vi "Configure.vi"(8 "error in (no error)":errorcluster, 9 "Path":path, 10 "Interactive?":bool, 11 "XML Report In":refnum<class "XML Report.lvclass">) -> (0 "error out":errorcluster, 3 "XML Report Out":refnum<class "XML Report.lvclass">)   [LabVIEW 2020, in "XML Report.lvclass"]
uses:
  XML Report.lvclass
  XML Report.lvclass/XML Report.ctl
  Framework/Configuration Manager/Configuration Manager.lvclass
panel:
  in  "Cancel":bool
  in  "Commit":bool
  in  "Open New Reports":bool
  in  "Report Path":path
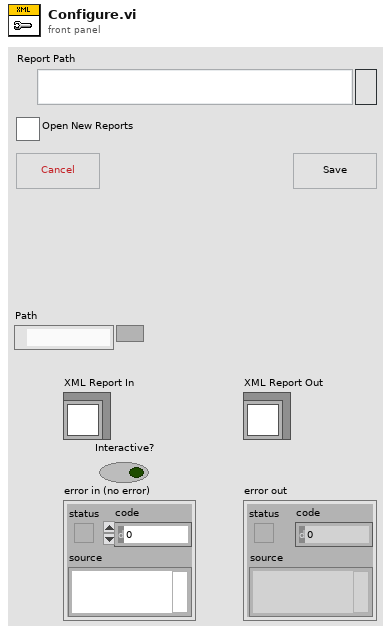
[diagram p1: front panel]
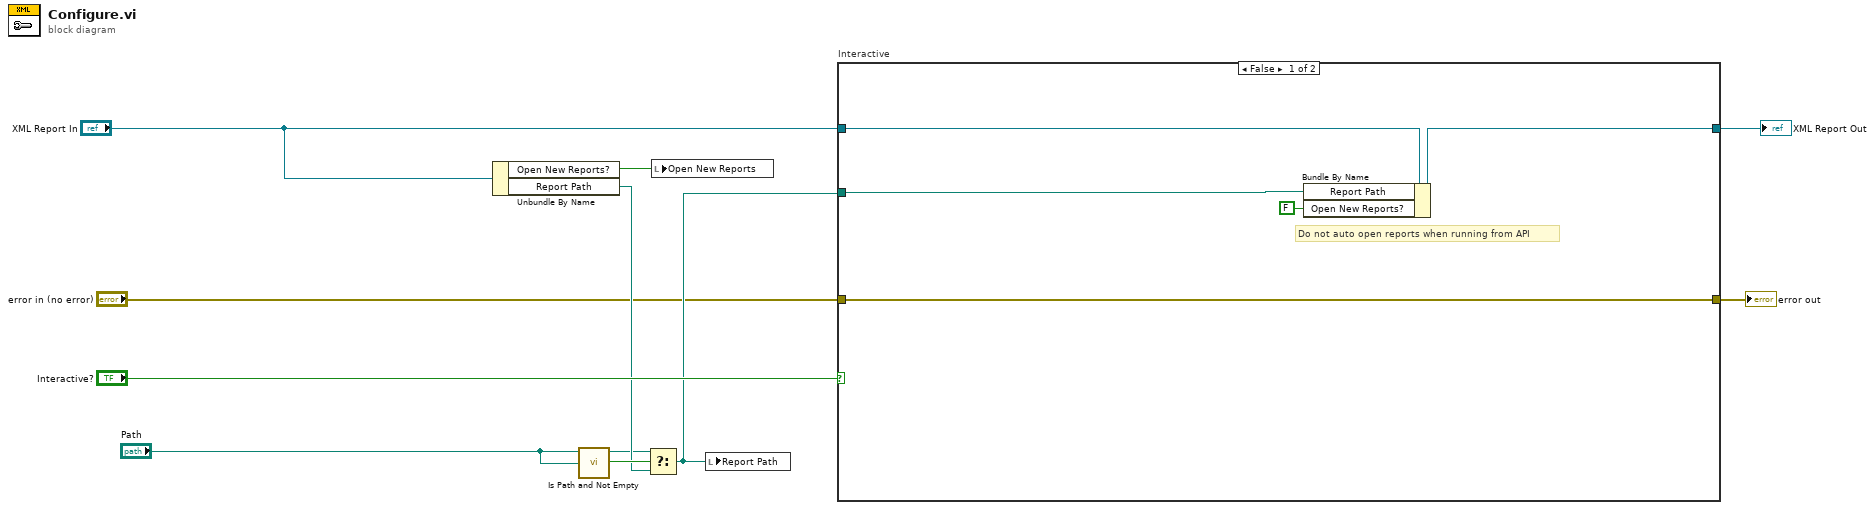
[diagram p0: block diagram]
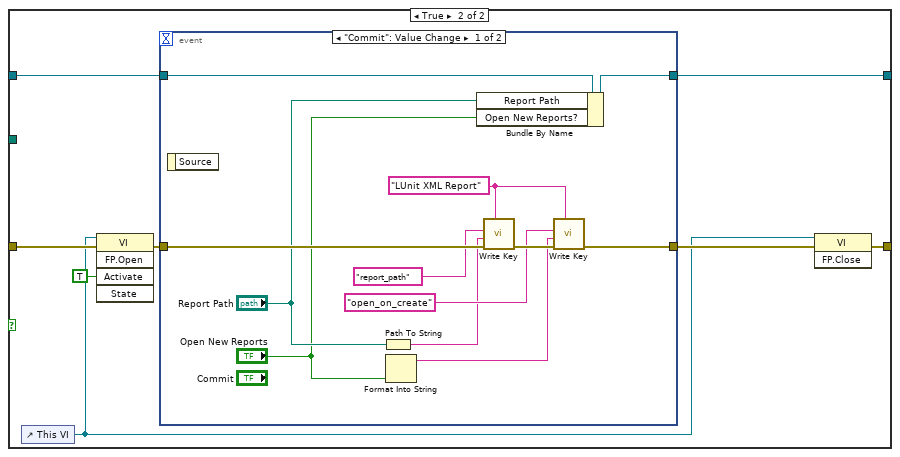
[diagram p2: hidden frame]
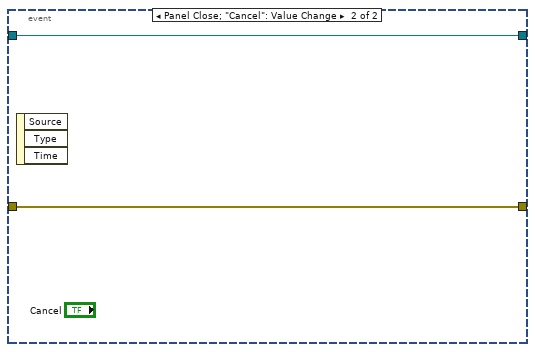
[diagram p3: hidden frame]
diagram:
  n1 = Unbundle By Name("XML Report In") -> ("Open New Reports?"=w4:bool, "Report Path"=w5:path)
  n2 = call <vilib>:"Is Path and Not Empty.vi"("path"="Path") -> ("Is Path and Not Empty?"=w6:bool)  [unwired: 4 in]
  n3 = Select(t="Path", s=w6, f=w5) -> (s? t:f=w7:path)
  n4 = local write "Open New Reports"(w4) -> ()
  n5 = local write "Report Path"(w7) -> ()
  n6 = case "Interactive" shown="False" "Interactive?" {
    tunnel: "error in (no error)" -> [w11 w21]
    tunnel: [w11 w19] -> w10
    tunnel: "XML Report In" -> [w13 w16]
    tunnel: [w15 w17] -> w8
    tunnel: w7 -> [w12 _]
    frame False {
      # "Do not auto open reports when running from API"
      n7 = Bundle By Name(cluster=w13, "Report Path"=w12, "Open New Reports?"=FALSE) -> (w15:refnum<class "XML Report.lvclass">)
    }
    frame True {
      n8 = control-ref of="This VI"() -> (w18:refnum<vi>)
      n9 = invoke class="VI" method="FP.Open"(reference=w18, error in=w21, "Activate"=TRUE ("Activate?")) -> (error out=w22:errorcluster)  [unwired: 2 in, 4 out]
      n10 = event shown="[0] \"Commit\": Value Change" {
        selector: _ -> [_ _]
        dyn-events: _ -> [_ _]
        timeout: _ -> [_ _]
        tunnel: w22 -> [w35 w37]
        tunnel: [w34 w37] -> w20
        tunnel: [w26 w36] -> w17
        tunnel: w16 -> [w27 w36]
        event "Commit": Value Change {
          w33 = "LUnit XML Report"
          n11 = event-data() -> ()  [unwired: 1 in, 1 out]
          n12 = Path To String(path="Report Path") -> (string=w29:string)
          n13 = Format Into String("Open New Reports") -> (resulting string=w28:string)  [unwired: 3 in, 1 out]
          n14 = Bundle By Name(cluster=w27, "Report Path"="Report Path", "Open New Reports?"="Open New Reports") -> (w26:refnum<class "XML Report.lvclass">)
          n15 = call "Write Key.vi"("section"=w33, "error in (no error)"=w35, "value"=w29, "key"="report_path" ("Name")) -> ("error out"=w32:errorcluster)  [unwired: 7 in]
          n16 = call "Write Key.vi"("section"=w33, "error in (no error)"=w32, "value"=w28, "key"="open_on_create" ("Name")) -> ("error out"=w34:errorcluster)  [unwired: 7 in]
        }
        event Panel Close; "Cancel": Value Change {
          n17 = event-data() -> ()  [unwired: 1 in, 3 out]
        }
      }
      n18 = invoke class="VI" method="FP.Close"(reference=w18, error in=w20) -> (error out=w19:errorcluster)  [unwired: 1 in, 2 out]
    }
  }
  "error out" <- w10
  "XML Report Out" <- w8
